vi "start client connect.vi"(5 "request id":u32, 6 "bufferMaxSize":u64=5242880, 7 "event":refnum<user-event>, 8 "error in":errorcluster, 9 "port":string, 10 "host":string, 11 "client":u64) -> (0 "error out":errorcluster)   [LabVIEW 2016, in "async tls dl.lvlib"]
uses:
  async tls dl.lvlib
  action complete event.ctl
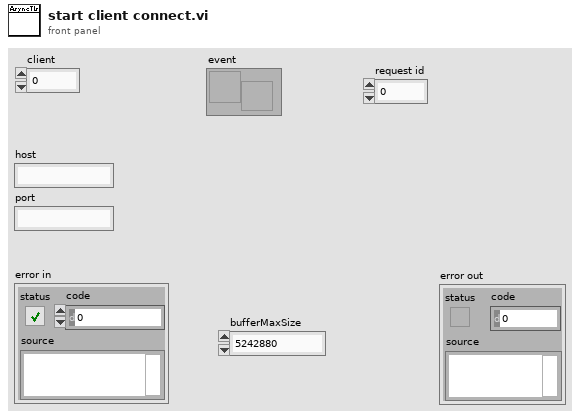
[diagram p1: front panel]
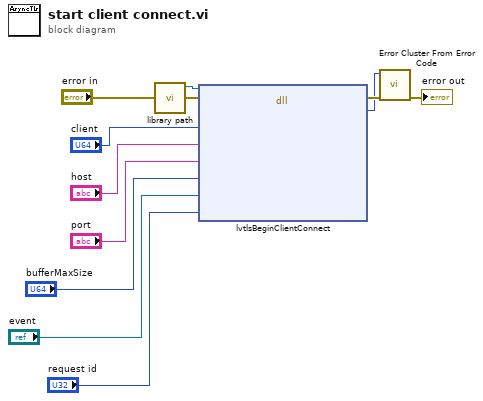
[diagram p0: block diagram]
diagram:
  n1 = call "library path.vi"() -> ("path"=w2:path)  [unwired: 11 in]
  n2 = dll-call lib="C:/Users/IEUser/Desktop/libasynclvtls/lvasynctls.dll" fn="lvtlsBeginClientConnect"(path in=w2, error in="error in", "client"="client", "host"="host", "port"="port", "bufferMaxSize"="bufferMaxSize", "event"="event", "id"="request id") -> (error out=w10:errorcluster, "err"=w9:i32)  [unwired: 7 in, 1 out]
  n3 = call <vilib>:"Error Cluster From Error Code.vi"("error in (no error)"=w10, "error code (0)"=w9) -> ("error out"=→"error out":errorcluster)  [unwired: 7 in]
